vi "Read Switching Function Status.vi"(8 "error in (no error)":errorcluster, 11 "VGC in":refnum<class "PL Inficon VGC.lvclass">) -> (0 "error out":errorcluster, 2 "status":bool[](array[boolean]), 3 "VGC out":refnum<class "PL Inficon VGC.lvclass">)   [LabVIEW 2015, in "PL Inficon VGC.lvclass"]
doc: "Reads switching funcion status."
uses:
  PL Inficon VGC.lvclass
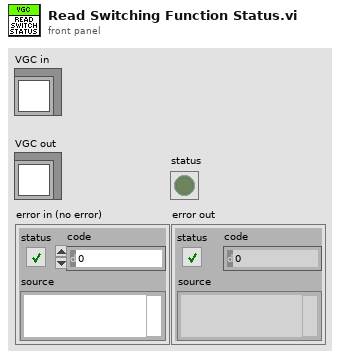
[diagram p1: front panel]
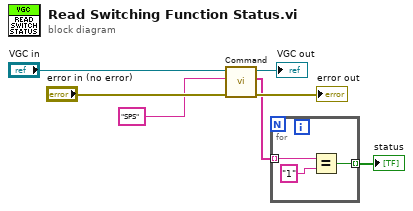
[diagram p0: block diagram]
diagram:
  n1 = call "Command.vi"("error in (no error)"="error in (no error)", "command"="SPS", "VGC in"="VGC in") -> ("error out"=→"error out":errorcluster, "response data"=w2:string[], "VGC out"=→"VGC out":refnum<class "PL Inficon VGC.lvclass">)  [unwired: 6 in]
  n2 = for {
    tunnel: w2 -> [w8] mode=indexing
    tunnel: [w9] -> w1 mode=indexing
    n3 = Equal?(x=w8, y="1") -> (x = y?=w9:bool)
  }
  "status" <- w1
